vi "Waiting rotate 2D (SubVI).vi"(3 "error in (no error)":errorcluster, 5 "VISA Refnum in":refnum<visa-resource-name>) -> (0 "error out":errorcluster)   [LabVIEW 2018]
uses:
  GlobalStop.vi
panel:
  out "Data?":bool
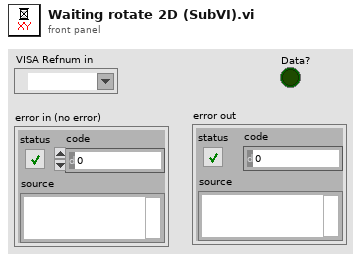
[diagram p1: front panel]
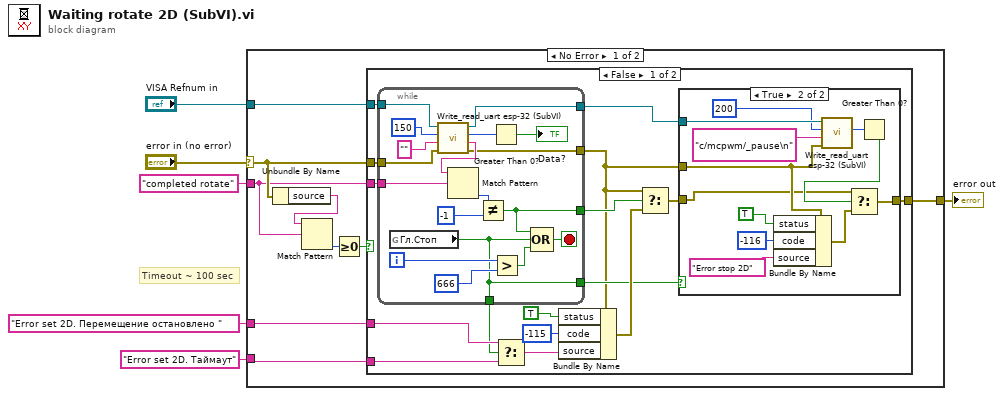
[diagram p0: block diagram]
diagram:
  # "Timeout ~ 100 sec"
  n1 = case shown="No Error" "error in (no error)" {
    selector: "error in (no error)" -> [w11 w64]
    tunnel: "completed rotate" -> [w10 _]
    tunnel: "VISA Refnum in" -> [w15 _]
    tunnel: "Error set 2D. Перемещение остановлено " -> [w14 _]
    tunnel: "Error set 2D. Таймаут" ("f") -> [w13 _]
    tunnel: [w12 w64] -> w2
    frame No Error {
      n2 = Unbundle By Name(w11) -> ("source"=w7:string)
      n3 = Match Pattern(string=w7, regular expression=w10) -> (offset past match=w8:i32)  [unwired: 1 in, 3 out]
      n4 = Greater Or Equal To 0?(x=w8) -> (x >= 0?=w9:bool)
      n5 = case shown="False" w9 {
        tunnel: w10 -> [w31 _]
        tunnel: w15 -> [w30 _]
        tunnel: w14 -> [w27 _]
        tunnel: w13 -> [w24 _]
        tunnel: [w18 w63] -> w12
        tunnel: w11 -> [w16 w63]
        frame False {
          n6 = while {
            tunnel: w31 -> [w56]
            tunnel: w16 -> [w55]
            tunnel: [w54] -> w17
            tunnel: w30 -> [w51]
            tunnel: [w50] -> w29
            tunnel: [w46] -> w26
            tunnel: [w46] -> w22
            tunnel: [w45] -> w19
            i -> [w49]
            stop <- w57 stop-if-true
            n7 = global read "GlobalStop.vi" "Гл.Стоп"() -> (w46:bool)
            n8 = call "Write_read_uart esp-32 (SubVI).vi"("error in (no error)"=w55, "write buffer"="", "milliseconds to wait"=u32 150, "VISA Refnum in"=w51) -> ("error out 4"=w54:errorcluster, "read buffer"=w60:string, "read bite"=w53:u32, "VISA resource name out"=w45:refnum<visa-resource-name>)
            n9 = Match Pattern(string=w60, regular expression=w56) -> (offset past match=w58:i32)  [unwired: 1 in, 3 out]
            n10 = Not Equal?(x=w58, y=-1 ("offset past match")) -> (x != y?=w50:bool)
            n11 = Greater Than 0?(x=w53) -> (x > 0?=→"Data?":bool)
            n12 = Greater?(x=w49, y=666) -> (0:w47:bool)
            n13 = Compound Arithmetic op=OR(w50, w46, w47) -> (w57:bool)
          }
          n14 = Select(t=w27, s=w26, f=w24) -> (s? t:f=w25:string)
          n15 = Bundle By Name(cluster=w17, "status"=TRUE, "code"=i16 -115, "source"=w25) -> (w23:errorcluster)
          n16 = Select(t=w17, s=w29, f=w23) -> (s? t:f=w21:errorcluster)
          n17 = case shown="True" w22 {
            tunnel: w21 -> [w32 w33]
            tunnel: w19 -> [_ w44]
            tunnel: [w32 w39] -> w18
            tunnel: w17 -> [_ w34]
            frame False {
            }
            frame True {
              n18 = Bundle By Name(cluster=w34, "status"=TRUE, "code"=i16 -116, "source"="Error stop 2D") -> (w35:errorcluster)
              n19 = call "Write_read_uart esp-32 (SubVI).vi"("error in (no error)"=w34, "write buffer"="c/mcpwm/_pause\n", "milliseconds to wait"=u32 200, "VISA Refnum in"=w44) -> ("read bite"=w41:u32)  [unwired: 3 out]
              n20 = Greater Than 0?(x=w41) -> (x > 0?=w40:bool)
              n21 = Select(t=w33, s=w40, f=w35) -> (s? t:f=w39:errorcluster)
            }
          }
        }
        frame True {
        }
      }
    }
    frame Error {
    }
  }
  "error out" <- w2
